vi "Windows Host.vi"() -> ()   [LabVIEW 2012]
uses:
  <vilib>/rvi/interface/RandomDataEmulation/nirviRandomDataOpen.vi
  <vilib>/rvi/interface/RandomDataEmulation/nirviRandomDataDMAMethods.vi
  <vilib>/rvi/interface/RandomDataEmulation/nirviRandomDataClose.vi
  <vilib>/rvi/interface/nirviOpenFPGA/nirviOpenFPGA.xnode
  FPGA Host.vi
  <vilib>/rvi/interface/nirviMethod/nirviMethod.xnode
  <vilib>/rvi/interface/nirviCloseFPGA/nirviCloseFPGA.xnode
panel:
  out "Data from FPGA":i16[](array[numeric])
  out "Empty Elements Remaining":u32
  in  "stop":bool
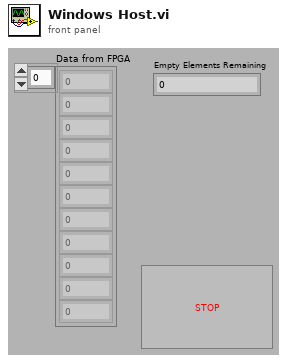
[diagram p1: front panel]
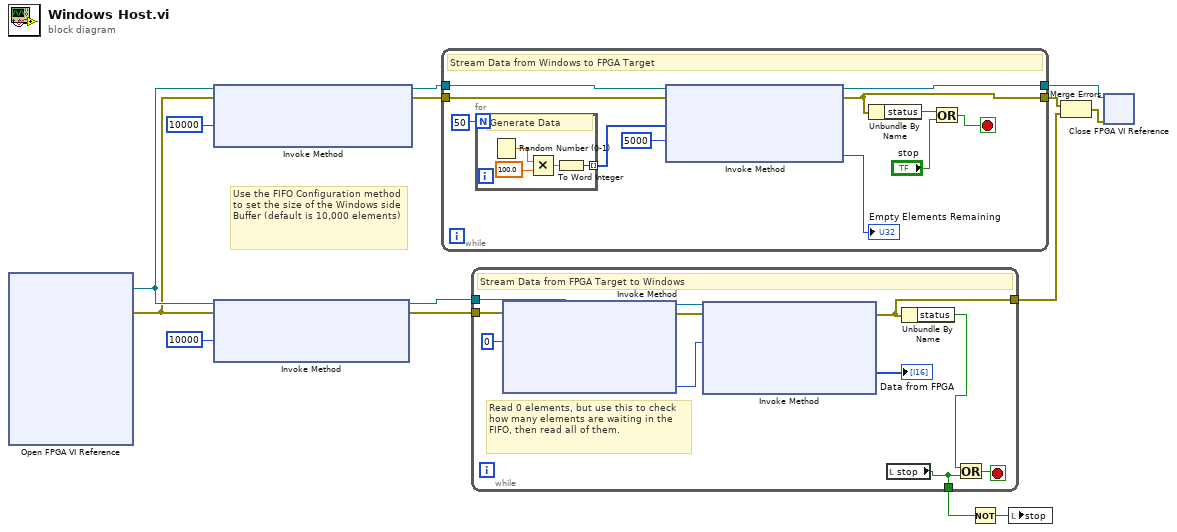
[diagram p0: block diagram]
diagram:
  # "Use the FIFO Configuration method to set the size of the Windows side Buffer (default is 10,000 elements)"
  n1 = xnode "Open FPGA VI Reference"() -> ("FPGA VI Reference Out"=w14:refnum<k20>, "error out"=w3:errorcluster)  [unwired: 2 in]
  n2 = xnode "Invoke Method"("FPGA VI Reference In"=w14, "error in"=w3, "Requested Depth"=u32 10000 ("Depth")) -> ("FPGA VI Reference Out"=w11:refnum<k20>, "error out"=w10:errorcluster)  [unwired: 1 out]
  n3 = xnode "Invoke Method"("FPGA VI Reference In"=w14, "error in"=w3, "Requested Depth"=u32 10000 ("Depth")) -> ("FPGA VI Reference Out"=w9:refnum<k20>, "error out"=w8:errorcluster)  [unwired: 1 out]
  n4 = while {
    tunnel: w11 -> [w25]
    tunnel: w10 -> [w24]
    tunnel: [w23] -> w7
    tunnel: [w20] -> w6
    stop <- w21 stop-if-true
    # "Stream Data from Windows to FPGA Target"
    n5 = for {
      N: 50 -> [_]
      tunnel: [w28] -> w16 mode=indexing
      # "Generate Data"
      n6 = Random Number (0-1)() -> (number: 0 to 1=w29:dbl)
      n7 = Multiply(x=w29, y=100.0) -> (x*y=w27:dbl)
      n8 = To Word Integer(number=w27) -> (16bit integer=w28:i16)
    }
    n9 = xnode "Invoke Method"("FPGA VI Reference In"=w25, "error in"=w24, "Data"=w16, "Timeout (ms)"=5000) -> ("FPGA VI Reference Out"=w23:refnum<k20>, "error out"=w20:errorcluster, "Empty Elements Remaining"=→"Empty Elements Remaining":u32)
    n10 = Unbundle By Name(w20) -> ("status"=w19:bool)
    n11 = Or(x=w19, y="stop") -> (x .or. y?=w21:bool)
  }
  n12 = while {
    tunnel: w9 -> [w40]
    tunnel: w8 -> [w39]
    tunnel: [w32] -> w5
    tunnel: [w30] -> w2
    stop <- w38 stop-if-true
    # "Read 0 elements, but use this to check how many elements are waiting in the FIFO, then read all of them."
    # "Stream Data from FPGA Target to Windows"
    n13 = xnode "Invoke Method"("FPGA VI Reference In"=w40, "error in"=w39, "Number of Elements"=u32 0) -> ("FPGA VI Reference Out"=w36:refnum<k20>, "error out"=w35:errorcluster, "Elements Remaining"=w34:u32)  [unwired: 1 in, 1 out]
    n14 = xnode "Invoke Method"("FPGA VI Reference In"=w36, "error in"=w35, "Number of Elements"=w34) -> ("error out"=w32:errorcluster, "Data"=→"Data from FPGA":i16[])  [unwired: 1 in, 2 out]
    n15 = local read "stop"() -> (w30:bool)
    n16 = Unbundle By Name(w32) -> ("status"=w31:bool)
    n17 = Or(x=w31, y=w30) -> (x .or. y?=w38:bool)
  }
  n18 = Not(x=w2) -> (.not. x?=w1:bool)
  n19 = local write "stop"(w1) -> ()
  n20 = Merge Errors(w6, w5) -> (w4:errorcluster)
  n21 = xnode "Close FPGA VI Reference"("FPGA VI Reference In"=w7, "error in"=w4) -> ()  [unwired: 1 out]
